vi "Load VRML File.vi"(8 "error in":errorcluster, 11 "Path":path) -> (0 "error out":errorcluster, 3 "Scene:Read Scene File":refnum<vi>)   [LabVIEW 2017, in "NI_3D Picture Control.lvlib"]
doc: "Loads a three-dimensional object model saved in Virtual Reality Modeling Language (VRML) format to display in a 3D scene. VRML files commonly appear with a .wrl file extension."
uses:
  <vilib>/picture/3D Picture Control/NI_3D Picture Control.lvlib
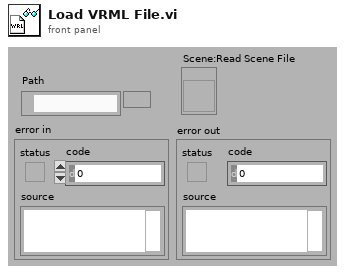
[diagram p1: front panel]
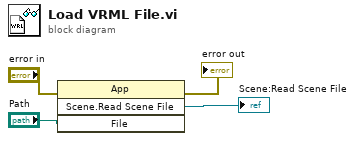
[diagram p0: block diagram]
diagram:
  n1 = invoke class="App" method="Scene.Read Scene File"(error in="error in", "File"="Path") -> (error out=→"error out":errorcluster, "Scene.Read Scene File"=→"Scene:Read Scene File":refnum<vi>)  [unwired: 2 in, 2 out]
